vi "close.vi"(8 "error in":errorcluster, 11 "SystemLin Tag Module runtime in":refnum<class "SystemLink runtime.lvclass">) -> (0 "error out":errorcluster)   [LabVIEW 2015, in "SystemLink runtime.lvclass"]
doc: "Provides an interface for terminating a module instance. While this interface performs no operations, a child should close and deallocate any open references or memory."
uses:
  SystemLink runtime.lvclass
  SystemLink runtime.lvclass/SystemLink runtime.ctl
  <vilib>/Skyline/Tag/Wrapper/Wrapper_class/Close Tag (Single).vi
  <vilib>/Skyline/Tag/Wrapper/Wrapper_class/NI Skyline Tag.lvclass
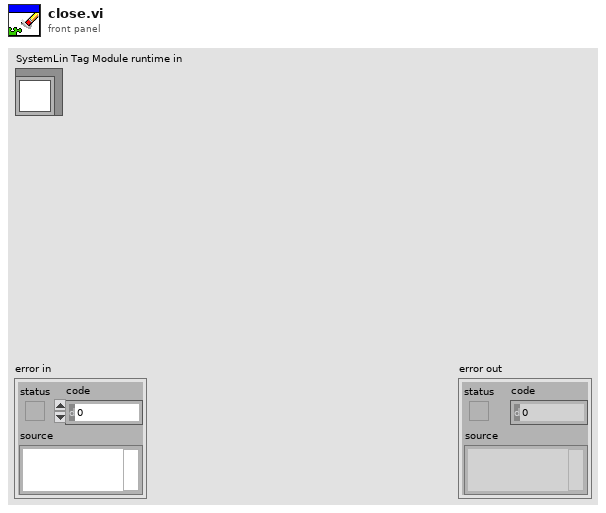
[diagram p1: front panel]
types:
  T1 = typedef "SystemLink configuration.lvclass/SysLink Mapping.ctl" = cluster{"Data Type":T2, "Tag Reference":refnum<class "NI Skyline Tag.lvclass">, "Tag Bus Index":i32, "AMQP":bool, "Skylink Index":i32}
  T2 = typedef "tag bus.lvlib/tag descriptor.lvclass/Data Type.ctl" = enum16{"Double", "Single", "I64", "I32", "I16", "I8", "U64", "U32", "U16", "U8", "Boolean", "String", "Array of Double", "Array of Single", "Array of I64", "Array of I32", "Array of I16", "Array of I8", "Array of U64", "Array of U32", "Array of U16", "Array of U8", "Array of Boolean", "Array of String"}
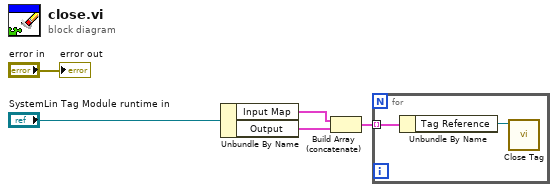
[diagram p0: block diagram]
diagram:
  n1 = Unbundle By Name("SystemLin Tag Module runtime in") -> ("Input Map"=w4:T1[], "Output"=w3:T1[])
  n2 = Build Array (concatenate)(w4, w3) -> (w2:T1[])
  n3 = for {
    tunnel: w2 -> [w7] mode=indexing
    n4 = Unbundle By Name(w7) -> ("Tag Reference"=w6:refnum<class "NI Skyline Tag.lvclass">)
    n5 = call-poly <vilib>:"Close Tag.vi"("tag in"=w6) -> ()  [unwired: 10 in, 1 out]
  }
  "error out" <- "error in"
